vi "Requirement Coverage.vi"() -> ()   [LabVIEW 2013]
uses:
  <vilib>/addons/_JKI Toolkits/Caraya/classes/Test/Test.lvclass
panel:
  out "error out":errorcluster
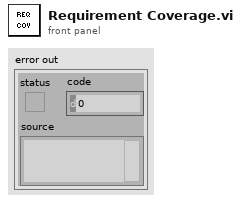
[diagram p1: front panel]
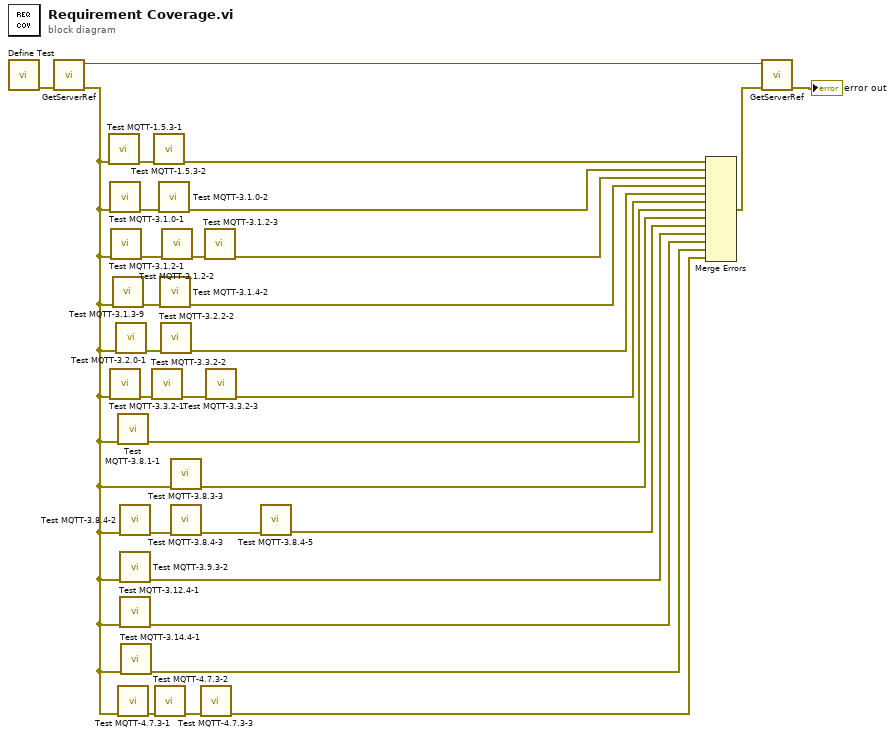
[diagram p0: block diagram]
diagram:
  n1 = call <vilib>:"Define Test.vi"() -> ("error out"=w25:errorcluster)  [unwired: 11 in]
  n2 = call "GetServerRef.vi"("error in"=w25) -> ("error out"=w3:errorcluster, "Created"=w24:bool)  [unwired: 8 in, 1 out]
  n3 = call "Test MQTT-1.5.3-1.vi"("error in (no error)"=w3) -> ("error out"=w15:errorcluster)  [unwired: 10 in]
  n4 = call "Test MQTT-3.1.0-1.vi"("error in (no error)"=w3) -> ("error out"=w26:errorcluster)  [unwired: 10 in]
  n5 = call "Test MQTT-3.3.2-1.vi"("error in (no error)"=w3) -> ("error out"=w16:errorcluster)  [unwired: 10 in]
  n6 = call "Test MQTT-3.1.2-1.vi"("error in (no error)"=w3) -> ("error out"=w28:errorcluster)  [unwired: 10 in]
  n7 = call "Test MQTT-3.1.3-9.vi"("error in (no error)"=w3) -> ("error out"=w29:errorcluster)  [unwired: 10 in]
  n8 = call "Test MQTT-3.2.0-1.vi"("error in (no error)"=w3) -> ("error out"=w27:errorcluster)  [unwired: 10 in]
  n9 = call "Test MQTT-3.8.1-1.vi"("error in (no error)"=w3) -> ("error out"=w14:errorcluster)  [unwired: 10 in]
  n10 = call "Test MQTT-4.7.3-1.vi"("error in (no error)"=w3) -> ("error out"=w4:errorcluster)  [unwired: 10 in]
  n11 = call "Test MQTT-3.8.4-2.vi"("error in (no error)"=w3) -> ("error out"=w9:errorcluster)  [unwired: 10 in]
  n12 = call "Test MQTT-3.9.3-2.vi"("error in (no error)"=w3) -> ("error out"=w11:errorcluster)  [unwired: 10 in]
  n13 = call "Test MQTT-3.12.4-1.vi"("error in (no error)"=w3) -> ("error out"=w7:errorcluster)  [unwired: 10 in]
  n14 = call "Test MQTT-3.14.4-1.vi"("error in (no error)"=w3) -> ("error out"=w5:errorcluster)  [unwired: 10 in]
  n15 = call "Test MQTT-3.3.2-2.vi"("error in (no error)"=w16) -> ("error out"=w13:errorcluster)  [unwired: 10 in]
  n16 = call "Test MQTT-1.5.3-2.vi"("error in (no error)"=w15) -> ("error out"=w21:errorcluster)  [unwired: 10 in]
  n17 = call "Test MQTT-4.7.3-2.vi"("error in (no error)"=w4) -> ("error out"=w2:errorcluster)  [unwired: 10 in]
  n18 = call "Test MQTT-3.1.0-2.vi"("error in (no error)"=w26) -> ("error out"=w20:errorcluster)  [unwired: 10 in]
  n19 = call "Test MQTT-3.1.4-2.vi"("error in (no error)"=w29) -> ("error out"=w18:errorcluster)  [unwired: 10 in]
  n20 = call "Test MQTT-3.2.2-2.vi"("error in (no error)"=w27) -> ("error out"=w17:errorcluster)  [unwired: 10 in]
  n21 = call "Test MQTT-3.1.2-2.vi"("error in (no error)"=w28) -> ("error out"=w30:errorcluster)  [unwired: 10 in]
  n22 = call "Test MQTT-3.8.3-3.vi"("error in (no error)"=w3) -> ("error out"=w6:errorcluster)  [unwired: 10 in]
  n23 = call "Test MQTT-3.8.4-3.vi"("error in (no error)"=w9) -> ("error out"=w8:errorcluster)  [unwired: 10 in]
  n24 = call "Test MQTT-4.7.3-3.vi"("error in (no error)"=w2) -> ("error out"=w1:errorcluster)  [unwired: 10 in]
  n25 = call "Test MQTT-3.1.2-3.vi"("error in (no error)"=w30) -> ("error out"=w19:errorcluster)  [unwired: 10 in]
  n26 = call "Test MQTT-3.3.2-3.vi"("error in (no error)"=w13) -> ("error out"=w10:errorcluster)  [unwired: 10 in]
  n27 = call "Test MQTT-3.8.4-5.vi"("error in (no error)"=w8) -> ("error out"=w12:errorcluster)  [unwired: 10 in]
  n28 = Merge Errors(w21, w20, w19, w18, w17, w10, w14, w6, w12, w11, w7, w5, w1) -> (w23:errorcluster)
  n29 = call "GetServerRef.vi"("error in"=w23, "Destroy (F)"=w24) -> ("error out"=→"error out":errorcluster)  [unwired: 7 in, 2 out]
